vi "Read tecEn.vi"(8 "error in":errorcluster, 11 "cPAS in":refnum<class "cPAS.lvclass">) -> (0 "error out":errorcluster, 2 "tecEn":refnum<k21>="Filter In", 3 "cPAS out":refnum<class "cPAS.lvclass">)   [LabVIEW 2015, in "cPAS.lvclass"]
uses:
  cPAS.lvclass
  cPAS.lvclass/cPAS.ctl
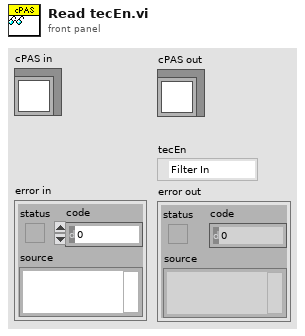
[diagram p1: front panel]
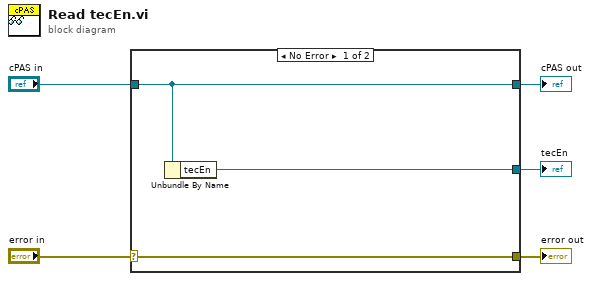
[diagram p0: block diagram]
diagram:
  n1 = case shown="No Error" "error in" {
    selector: "error in" -> [w8 w9]
    tunnel: [w8 w9] -> w4
    tunnel: [w7 w10] -> w2
    tunnel: "cPAS in" -> [w7 w10]
    tunnel: [w6 _] -> w1
    frame No Error {
      n2 = Unbundle By Name(w7) -> ("tecEn"=w6:refnum<k21>)
    }
    frame Error {
    }
  }
  "error out" <- w4
  "cPAS out" <- w2
  "tecEn" <- w1
